vi "Error 5006 - ProtoBuf Message Could Not Be Decoded.vi"() -> (0 "error out":errorcluster)   [LabVIEW 2020]
doc: "Error 5006 - ProtoBuf Message Could Not Be Decoded"
uses:
  <vilib>/Utility/error.llb/Error Cluster From Error Code.vi
  <vilib>/ErrorRing/Error Ring.xnode
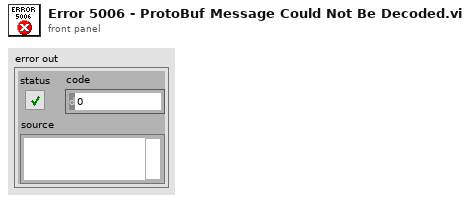
[diagram p1: front panel]
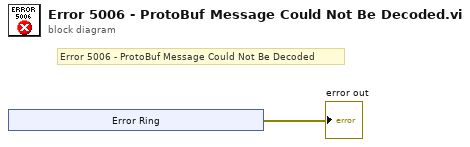
[diagram p0: block diagram]
diagram:
  # "Error 5006 - ProtoBuf Message Could Not Be Decoded"
  n1 = xnode "Error Ring"() -> ("error out"=→"error out":errorcluster)
